vi "Read Key Value String.vi"(7 "Section Name":string, 8 "error in (no error)":errorcluster, 9 "Default":string, 10 "Key Name":string, 11 "ODBC-Interface in":refnum<class "ODBC-Interface.lvclass">) -> (0 "error out":errorcluster, 1 "Value":string, 2 "found":bool, 3 "ODBC-Interface out":refnum<class "ODBC-Interface.lvclass">)   [LabVIEW 2014, in "DB-Configuration.lvlib" / "ODBC-Interface.lvclass"]
doc: "Read string key value."
uses:
  ODBC-Interface.lvclass
  <vilib>/addons/database/_DB Variant To Data/Database Variant To Data.xnode
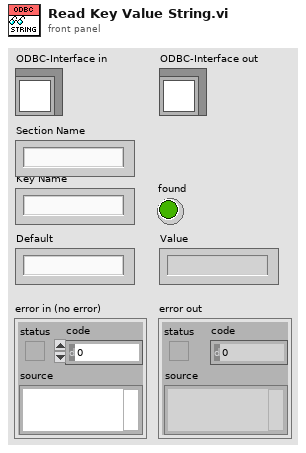
[diagram p1: front panel]
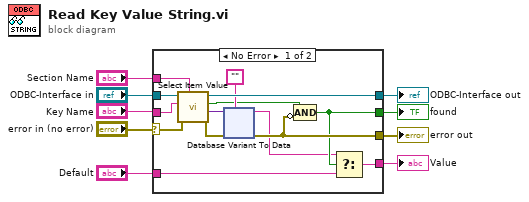
[diagram p0: block diagram]
diagram:
  n1 = case shown="No Error" "error in (no error)" {
    selector: "error in (no error)" -> [w11 w57]
    tunnel: "ODBC-Interface in" -> [w23 w58]
    tunnel: [w22 w58] -> w4
    tunnel: "Section Name" -> [w21 _]
    tunnel: "Key Name" -> [w20 _]
    tunnel: [w15 w57] -> w2
    tunnel: [w14 _] -> w3
    tunnel: [w13 w56] -> w1
    tunnel: "Default" -> [w12 w56]
    frame No Error {
      n2 = call-dynamic "Select Item Value.vi"("Section Name"=w21, "error in (no error)"=w11, "Key Name"=w20, "ODBC-Interface in"=w23) -> ("error out"=w18:errorcluster, "Value"=w19:variant, "found"=w16:bool, "ODBC-Interface out"=w22:refnum<class "ODBC-Interface.lvclass">)  [unwired: 4 in]
      n3 = xnode "Database Variant To Data"("database variant"=w19, "error in (no error)"=w18, "type"="") -> ("data"=w10:string, "error out"=w15:errorcluster)
      n4 = Compound Arithmetic op=AND(w16, invert w15) -> (w14:bool)
      n5 = Select(t=w10, s=w14, f=w12) -> (s? t:f=w13:string)
    }
    frame Error {
    }
  }
  "error out" <- w2
  "ODBC-Interface out" <- w4
  "Value" <- w1
  "found" <- w3
